vi "Stop Core.vi"(10 "final error code":i32, 11 "Software Lock-in in":refnum<class "Software Lock-in.lvclass">) -> (3 "Software Lock-in out":refnum<class "Software Lock-in.lvclass">)   [LabVIEW 2015, in "Software Lock-in.lvclass"]
doc: "(<B>Filename</B>: Actor Framework.lvlib:Actor.lvclass:Stop Core.vi)\n\nDefines what the actor does before it stops. Use the <B>final error code</B> input to determine whether the actor shut down in response to an error.\n\nBy default, this method does nothing. A descendant class may override it to define behavior, such as shutting down any processes the actor initiated in its override of the Actor Core method."
uses:
  Software Lock-in.lvclass
  Software Lock-in.lvclass/Software Lock-in.ctl
  Mag Lab Hardware.lvclass
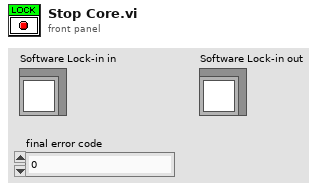
[diagram p1: front panel]
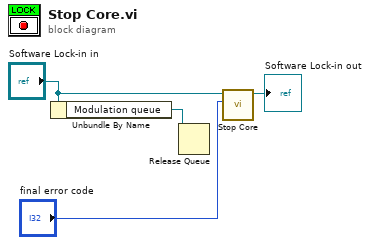
[diagram p0: block diagram]
diagram:
  n1 = Unbundle By Name("Software Lock-in in") -> ("Modulation queue"=w1:refnum<queue>)
  n2 = Release Queue(queue=w1) -> ()  [unwired: 2 in, 3 out]
  n3 = call-parent "Stop Core.vi"("final error code"="final error code", "Mag Lab Measure Base in"="Software Lock-in in") -> ("Mag Lab Measure Base out"=→"Software Lock-in out":refnum<class "Software Lock-in.lvclass">)  [unwired: 9 in]
